vi "Send SET Command.vi"(8 "error in (no error)":errorcluster, 9 "Control Value":variant, 10 "Control Name":string, 11 "TCP Network Connection in":refnum<k5>) -> (0 "error out":errorcluster)   [LabVIEW 2021]
doc: "Author: Scott Hannahs <sth@magnet.fsu.edu>\nCopyright 2018 Florida State University, All rights reserved."
uses:
  SCM4 Interlock/RT SubVIs/Interlock 32T FPGA Configure Parameters.ctl
  <vilib>/Utility/error.llb/Error Cluster From Error Code.vi
  TCP Functions/TCP Write Length and Data (I16).vi
  TCP Functions/TCP Write Length and Data (U16).vi
  TCP Functions/TCP Write Length and Data (I32).vi
  TCP Functions/TCP Write Length and Data (U32).vi
  TCP Functions/TCP Write Length and Data (DBL).vi
  TCP Functions/TCP Write Length and Data (STR).vi
  TCP Functions/TCP Write Length and Data (Bool).vi
  TCP Functions/TCP Write Length and Data (Variant).vi
  TCP Functions/TCP Write Length and Data (Array I16).vi
  TCP Functions/TCP Write Length and Data (Array DBL).vi
  TCP Functions/TCP Write Length and Data (2D Array DBL).vi
  <vilib>/ErrorRing/Error Ring.xnode
  <vilib>/Utility/Data Type/NI_Data Type.lvlib
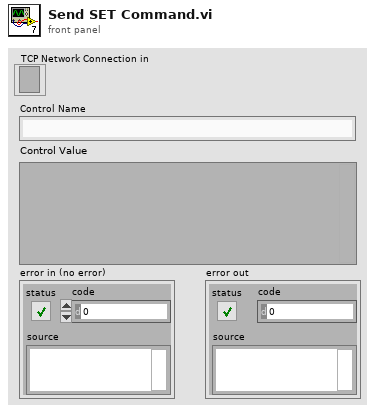
[diagram p1: front panel]
types:
  T1 = typedef "NI_Data Type.lvlib/Data Type.ctl" = enum8{"Invalid Type", "Void", "I8", "I16", "I32", "I64", "U8", "U16", "U32", "U64", "Single Float", "Double Float", "Extended Float", "Single Complex", "Double Complex", "Extended Complex", "Enum U8", "Enum U16", "Enum U32", "Enum U64", "Single Float With Unit", "Double Float With Unit", "Extended Float With Unit", "Single Complex with Unit", "Double Complex with Unit", "Extended Complex with Unit", "Boolean", "String", "Path", "Picture", "Tag", "Array", "Cluster", "Variant", "LV Variant", "Waveform", "Timestamp", "Digital Waveform", "Digital Data", "ExpressData", "Refnum", "External Data", "VI", "Poly VI", "LabVIEW Class Instance", "Fixed Point", "Set Collection", "Map Collection"}
  T2 = typedef "Interlock 32T FPGA Configure Parameters.ctl" = cluster{"Ch Scale":dbl[], "HTS Shunt Offset (V)":dbl, "LTS Shunt Offset (V)":dbl, "Crowbar Loop Time (ms)":u32, "Ramp To Zero Loop Time (mSec)":u32, "WDT Check Loop Ticks":u32, "Trip Threshold Currents":i16[], "Contactor OFF Current":dbl, "Contactor ON Current":dbl, "Quench Loop Thresh":dbl, "SW1 Vout Thresh":dbl, "HTS Current Mismatch":dbl, "LTS Current Mismatch":dbl, "DAQ Loop Timer (Ticks)":u32, "Crowbar Reset Countdown Length (ms)":i32, "Helium Low Levels":dbl, "# Low Readings":u32, "Battery Low Warn":dbl, "Notification Email":string, "Helium Level #1 VISA Resource":string, "Helium Level #2 VISA Resource":string, "LTS Power Supply Control":string, "HTS Power Supply Control":string, "Prologix GPIB Address":string, "LTS DMM GPIB":u32, "HTS DMM GPIB":u32, "Crowbar Unlock Safe Limit":dbl, "Logic PWR Thresh":dbl, "Batt Mon Read Timeout":i32, "Batt Mon Wait Timeout":i32, "Field Diff Max":dbl, "Field Diff Count":u16, "Contactor Closed Time (mS)":i32}
  T3 = cluster{"Ch Scale":dbl[], "HTS Shunt Offset (V)":dbl, "LTS Shunt Offset (V)":dbl, "Crowbar Loop Time (ms)":u32, "Ramp To Zero Loop Time (mSec)":u32, "WDT Check Loop Ticks":u32, "Trip Threshold Currents":i16[], "Contactor OFF Current":dbl, "Contactor ON Current":dbl, "Quench Loop Thresh":dbl, "SW1 Vout Thresh":dbl, "HTS Current Mismatch":dbl, "LTS Current Mismatch":dbl, "DAQ Loop Timer (Ticks)":u32, "Crowbar Reset Countdown Length (ms)":i32, "Helium Low Levels":dbl, "# Low Readings":u32, "Battery Low Warn":dbl, "Notification Email":string, "Helium Level #1 VISA Resource":string, "Helium Level #2 VISA Resource":string, "LTS Power Supply Control":string, "HTS Power Supply Control":string, "Prologix GPIB Address":string, "LTS DMM GPIB":u32, "HTS DMM GPIB":u32, "Crowbar Unlock Safe Limit":dbl, "Logic PWR Thresh":dbl, "Batt Mon Read Timeout":i32, "Batt Mon Wait Timeout":i32, "Field Diff Max":dbl, "Field Diff Count":u16, "Contactor Closed Time (mS)":i32}
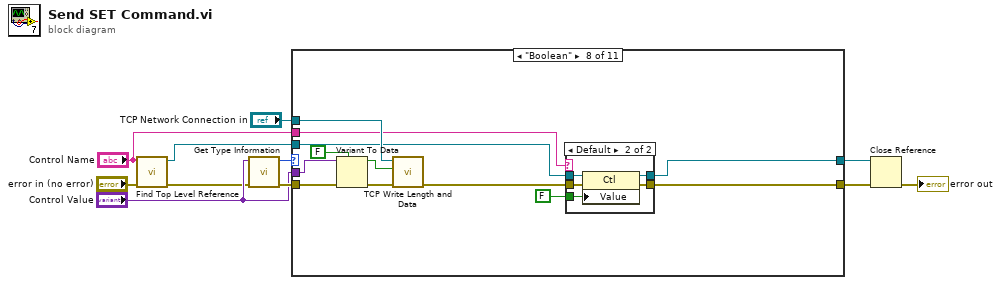
[diagram p0: block diagram]
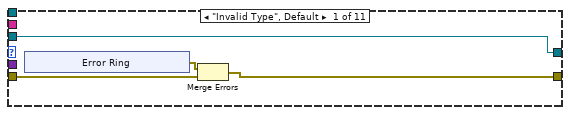
[diagram p2: hidden frame]
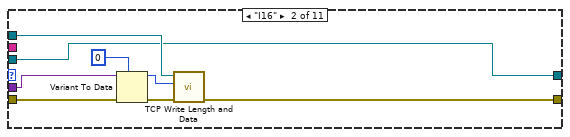
[diagram p3: hidden frame]
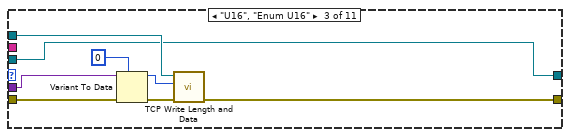
[diagram p4: hidden frame]
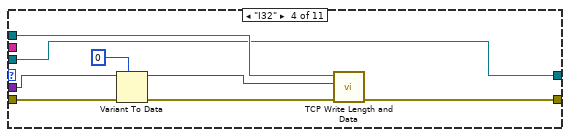
[diagram p5: hidden frame]
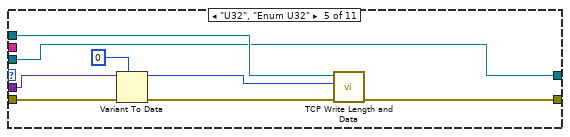
[diagram p6: hidden frame]
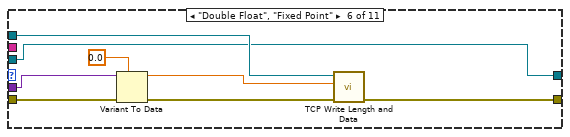
[diagram p7: hidden frame]
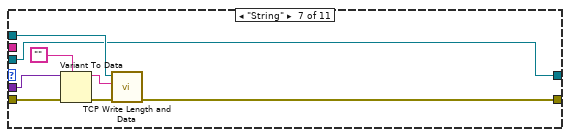
[diagram p8: hidden frame]
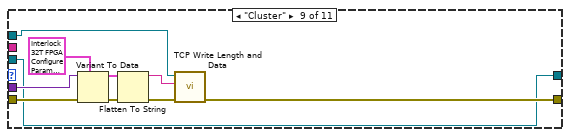
[diagram p10: hidden frame]
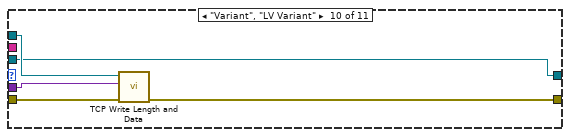
[diagram p11: hidden frame]
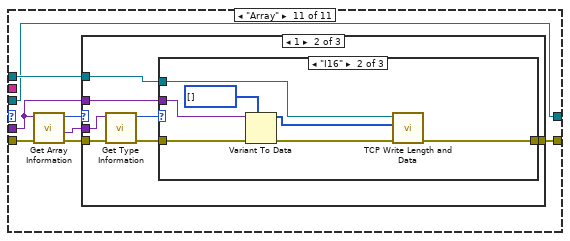
[diagram p12: hidden frame]
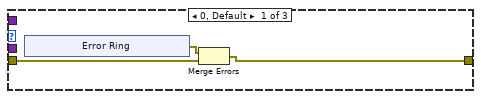
[diagram p13: hidden frame]
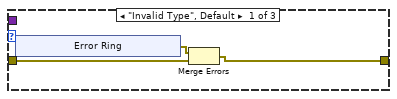
[diagram p14: hidden frame]
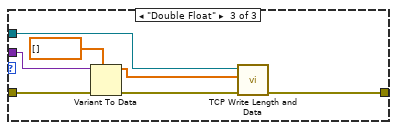
[diagram p15: hidden frame]
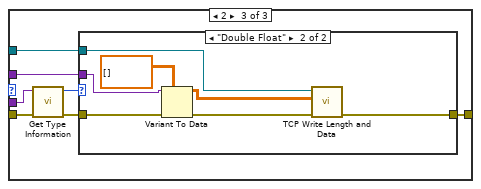
[diagram p16: hidden frame]
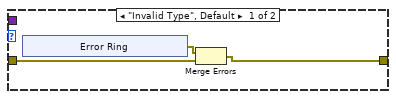
[diagram p17: hidden frame]
diagram:
  n1 = call "Find Top Level Reference.vi"("error in (no error)"="error in (no error)", "String"="Control Name") -> ("error out"=w1:errorcluster, "Ctl Refnum"=w11:refnum<vi>)  [unwired: 8 in]
  n2 = call <vilib>:"Get Type Information.vi"("error in (no error)"=w1, "variant"="Control Value") -> ("error out"=w10:errorcluster, "type"=w8:T1)  [unwired: 5 in, 3 out]
  n3 = case shown="\"Boolean\"" w8 {
    tunnel: "Control Value" -> [_ w28 w36 w44 w52 w60 w68 w80 w97 w100 w104]
    tunnel: "TCP Network Connection in" -> [_ w26 w34 w42 w50 w58 w66 w78 w96 w102 w110]
    tunnel: w10 -> [w15 w24 w32 w40 w48 w56 w64 w77 w95 w99 w106]
    tunnel: [w14 w22 w30 w38 w46 w54 w62 w74 w94 w101 w109] -> w5
    tunnel: w11 -> [w12 w21 w29 w37 w45 w53 w61 w73 w89 w98 w103]
    tunnel: "Control Name" -> [_ _ _ _ _ _ _ w70 _ _ _]
    tunnel: [w12 w21 w29 w37 w45 w53 w61 w69 w89 w98 w103] -> w3
    frame "Invalid Type", Default {
      n4 = xnode "Error Ring"() -> ("error out"=w13:errorcluster)
      n5 = Merge Errors(w13, w15) -> (w14:errorcluster)
    }
    frame "I16" {
      n6 = Variant To Data(error in=w24, type=i16 0, Variant=w28) -> (data=w25:i16, error out=w23:errorcluster)
      n7 = call-poly "TCP Write Length and Data.vi"("Error In"=w23, "Data"=w25, "connection ID"=w26) -> ("Error Out"=w22:errorcluster)  [unwired: 7 in, 1 out]
    }
    frame "U16", "Enum U16" {
      n8 = Variant To Data(error in=w32, type=i16 0, Variant=w36) -> (data=w33:i16, error out=w31:errorcluster)
      n9 = call-poly "TCP Write Length and Data.vi"("Error In"=w31, "Data"=w33, "connection ID"=w34) -> ("Error Out"=w30:errorcluster)  [unwired: 7 in, 1 out]
    }
    frame "I32" {
      n10 = Variant To Data(error in=w40, type=0, Variant=w44) -> (data=w41:i32, error out=w39:errorcluster)
      n11 = call-poly "TCP Write Length and Data.vi"("Error In"=w39, "Data"=w41, "connection ID"=w42) -> ("Error Out"=w38:errorcluster)  [unwired: 7 in, 1 out]
    }
    frame "U32", "Enum U32" {
      n12 = Variant To Data(error in=w48, type=u32 0, Variant=w52) -> (data=w49:u32, error out=w47:errorcluster)
      n13 = call-poly "TCP Write Length and Data.vi"("Error In"=w47, "Data"=w49, "connection ID"=w50) -> ("Error Out"=w46:errorcluster)  [unwired: 7 in, 1 out]
    }
    frame "Double Float", "Fixed Point" {
      n14 = Variant To Data(error in=w56, type=0.0, Variant=w60) -> (data=w57:dbl, error out=w55:errorcluster)
      n15 = call-poly "TCP Write Length and Data.vi"("Error In"=w55, "Data"=w57, "connection ID"=w58) -> ("Error Out"=w54:errorcluster)  [unwired: 7 in, 1 out]
    }
    frame "String" {
      n16 = Variant To Data(error in=w64, type="", Variant=w68) -> (data=w65:string, error out=w63:errorcluster)
      n17 = call-poly "TCP Write Length and Data.vi"("Error In"=w63, "Data"=w65, "connection ID"=w66) -> ("Error Out"=w62:errorcluster)  [unwired: 7 in, 1 out]
    }
    frame "Boolean" {
      n18 = Variant To Data(error in=w77, type=FALSE, Variant=w80) -> (data=w72:bool, error out=w76:errorcluster)
      n19 = call-poly "TCP Write Length and Data.vi"("Error In"=w76, "Data"=w72, "connection ID"=w78) -> ("Error Out"=w75:errorcluster)  [unwired: 7 in, 1 out]
      n20 = case shown="Default" w70 {
        tunnel: w75 -> [w82 w87]
        tunnel: [w82 w86] -> w74
        tunnel: w73 -> [w81 w85]
        tunnel: FALSE -> [_ w84]
        tunnel: [w81 w83] -> w69
        frame "Signal Injection On" {
        }
        frame Default {
          n21 = property class="Ctl"(reference=w85, error in=w87, "Value"=w84) -> (reference out=w83:refnum<vi>, error out=w86:errorcluster)
        }
      }
    }
    frame "Cluster" {
      n22 = Variant To Data(error in=w95, type=T2 {"Ch Scale"=[1.0, 1.0, 50.0, 20.0, 50.0, 30.0, 1.0, 200.0, 1.0, 1.0, 1.0, 1.0, 1.0], "HTS Shunt Offset (V)"=0.999969482421875, "LTS Shunt Offset (V)"=0.0, "Crowbar Loop Time (ms)"=512, "Ramp To Zero Loop Time (mSec)"=10, "WDT Check Loop Ticks"=40, "Trip Threshold Currents"=[0, 50, 50], "Contactor OFF Current"=1.0, "Contactor ON Current"=3.0, "Quench Loop Thresh"=1.5, "SW1 Vout Thresh"=15.0, "HTS Current Mismatch"=1.0, "LTS Current Mismatch"=1.0, "DAQ Loop Timer (Ticks)"=360, "Crowbar Reset Countdown Length (ms)"=10, "Helium Low Levels"=25.0, "# Low Readings"=3, "Battery Low Warn"=450.0, "Notification Email"="NHMFL DCFF Turnover <turnover@magnet.fsu.edu>", "Helium Level #1 VISA Resource"="TCPIP0::m1700-17-190::7180::SOCKET", "Helium Level #2 VISA Resource"="TCPIP0::m1700-17-191::7180::SOCKET", "LTS Power Supply Control"="TCPIP0::146.201.236.95::7180::SOCKET", "HTS Power Supply Control"="TCPIP0::146.201.236.94::7180::SOCKET", "Prologix GPIB Address"="tcpip::prologix-00-21-69-01-04-af.ad.magnet.fsu.edu::1234::socket", "LTS DMM GPIB"=23, "HTS DMM GPIB"=25, "Crowbar Unlock Safe Limit"=0.0, "Logic PWR Thresh"=1.0, "Batt Mon Read Timeout"=10000, "Batt Mon Wait Timeout"=130000, "Field Diff Max"=0.1, "Field Diff Count"=10, "Contactor Closed Time (mS)"=4096} ("Interlock 32T FPGA Configuration Values In"), Variant=w97) -> (data=w92:T3, error out=w91:errorcluster)
      n23 = Flatten To String(anything=w92, error in (no error)=w91) -> (data string=w93:string, error out=w90:errorcluster)  [unwired: 2 in, 1 out]
      n24 = call-poly "TCP Write Length and Data.vi"("Error In"=w90, "Data"=w93, "connection ID"=w96) -> ("Error Out"=w94:errorcluster)  [unwired: 7 in, 1 out]
    }
    frame "Variant", "LV Variant" {
      n25 = call-poly "TCP Write Length and Data.vi"("Error In"=w99, "Data"=w100, "connection ID"=w102) -> ("Error Out"=w101:errorcluster)  [unwired: 7 in, 1 out]
    }
    frame "Array" {
      n26 = call <vilib>:"Get Array Information.vi"("error in (no error)"=w106, "variant"=w104) -> ("error out"=w105:errorcluster, "array element data type"=w107:variant, "number of dimensions"=w108:i32)  [unwired: 6 in, 1 out]
      n27 = case shown="1" w108 {
        tunnel: w104 -> [_ w125 w154]
        tunnel: w110 -> [_ w124 w153]
        tunnel: w105 -> [w112 w120 w149]
        tunnel: [w111 w123 w152] -> w109
        tunnel: w107 -> [_ w122 w151]
        frame 0, Default {
          n28 = xnode "Error Ring"() -> ("error out"=w113:errorcluster)
          n29 = Merge Errors(w113, w112) -> (w111:errorcluster)
        }
        frame 1 {
          n30 = call <vilib>:"Get Type Information.vi"("error in (no error)"=w120, "variant"=w122) -> ("error out"=w119:errorcluster, "type"=w121:T1)  [unwired: 5 in, 3 out]
          n31 = case shown="\"I16\"" w121 {
            tunnel: w125 -> [_ w140 w147]
            tunnel: w124 -> [_ w139 w146]
            tunnel: w119 -> [w127 w137 w144]
            tunnel: [w126 w135 w142] -> w123
            frame "Invalid Type", Default {
              n32 = xnode "Error Ring"() -> ("error out"=w128:errorcluster)
              n33 = Merge Errors(w128, w127) -> (w126:errorcluster)
            }
            frame "I16" {
              n34 = Variant To Data(error in=w137, type=i16[] [], Variant=w140) -> (data=w138:i16[], error out=w136:errorcluster)
              n35 = call-poly "TCP Write Length and Data.vi"("Error In"=w136, "Data"=w138, "connection ID"=w139) -> ("Error Out"=w135:errorcluster)  [unwired: 7 in, 1 out]
            }
            frame "Double Float" {
              n36 = Variant To Data(error in=w144, type=dbl[] [], Variant=w147) -> (data=w145:dbl[], error out=w143:errorcluster)
              n37 = call-poly "TCP Write Length and Data.vi"("Error In"=w143, "Data"=w145, "connection ID"=w146) -> ("Error Out"=w142:errorcluster)  [unwired: 7 in, 1 out]
            }
          }
        }
        frame 2 {
          n38 = call <vilib>:"Get Type Information.vi"("error in (no error)"=w149, "variant"=w151) -> ("error out"=w148:errorcluster, "type"=w150:T1)  [unwired: 5 in, 3 out]
          n39 = case shown="\"Double Float\"" w150 {
            tunnel: w154 -> [_ w169]
            tunnel: w153 -> [_ w168]
            tunnel: w148 -> [w156 w166]
            tunnel: [w155 w164] -> w152
            frame "Invalid Type", Default {
              n40 = xnode "Error Ring"() -> ("error out"=w157:errorcluster)
              n41 = Merge Errors(w157, w156) -> (w155:errorcluster)
            }
            frame "Double Float" {
              n42 = Variant To Data(error in=w166, type=dbl[][] [], Variant=w169) -> (data=w167:dbl[][], error out=w165:errorcluster)
              n43 = call-poly "TCP Write Length and Data.vi"("Error In"=w165, "Data"=w167, "connection ID"=w168) -> ("Error Out"=w164:errorcluster)  [unwired: 7 in, 1 out]
            }
          }
        }
      }
    }
  }
  n44 = Close Reference(reference=w3, error in (no error)=w5) -> (error out=→"error out":errorcluster)
